vi "CAN Set Value.vi"   [LabVIEW 2020, in "PCANBasic.lvlib"]
uses:
  <userlib>/PCAN Basic/PCANBasic.lvlib
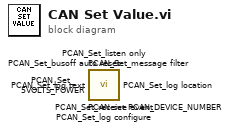
[diagram p0: block diagram]
diagram:
  n1 = call <userlib>:"PCAN_Set_receive event.vi"() -> ()  [unwired: 10 in, 2 out]
  n2 = call <userlib>:"PCAN_Set_message filter.vi"() -> ()  [unwired: 10 in, 2 out]
  n3 = call <userlib>:"PCAN_Set_log text.vi"() -> ()  [unwired: 10 in, 2 out]
  n4 = call <userlib>:"PCAN_Set_log location.vi"() -> ()  [unwired: 10 in, 2 out]
  n5 = call <userlib>:"PCAN_Set_log configure.vi"() -> ()  [unwired: 10 in, 2 out]
  n6 = call <userlib>:"PCAN_Set_listen only.vi"() -> ()  [unwired: 10 in, 2 out]
  n7 = call <userlib>:"PCAN_Set_busoff auto reset.vi"() -> ()  [unwired: 10 in, 2 out]
  n8 = call <userlib>:"PCAN_Set_5VOLTS_POWER.vi"() -> ()  [unwired: 10 in, 2 out]
  n9 = call <userlib>:"PCAN set PCAN_DEVICE_NUMBER.vi"() -> ()  [unwired: 10 in, 2 out]
